vi "_Main_ByRuns_DAC2022_V1.0.vi"() -> ()   [LabVIEW 2017]
uses:
  <vilib>/Instr/_visa.llb/VISA Configure Serial Port (Instr).vi
panel:
  out "Field, kV/cm":dbl
  out "Current, mA":dbl
  out "Voltage, V":dbl
  in  "COM DAC":refnum<visa-resource-name>
  in  "WaveForm":i32(listbox)
  in  "Auto\nturn OFF":bool
  in  "Content":i32(listbox)
  out "LastTrigTimer, s":dbl
  in  "Graph every, cycle":dbl=10.0 min=1.0 max=100.0
  in  "SendPeriod, ms":dbl=100.0 min=10.0 max=10000.0
  out "RunsNeed":i32
  out "Time LOG":cluster{dbl[], dbl[]}(graph)
  out "TrigTimer, s":dbl
  out "Bytes at Port":u32
  out "RecTry":i32
  out "OutVoltage, V":dbl
  in  "Exposition, s":dbl=3.0
  out "Channel 2, V":dbl format="%#_5g"
  out "Channel 1, V":dbl format="%#_5g"
  in  "Stop Button":bool
  in  "Start Button":bool
  in  "Sample H, um":dbl=32.0
  out "VoltageArray, V":dbl[](array[numeric])
  out "Shutter Red":bool
  out "Shutter Green":bool
  in  "Frames In Run":u32=180
  out "Global Frame Done":u32
  out "Now is Run #":u32
  out "Frame In Run Done":u32
  in  "Step, kV/cm":dbl=1.0 min=0.01 max=1000.0
  in  "Amplitude, kV/cm":dbl=10.0 min=10.0 max=1500.0
  in  "LOG file":path
  in  "COM ADC":refnum<visa-resource-name>
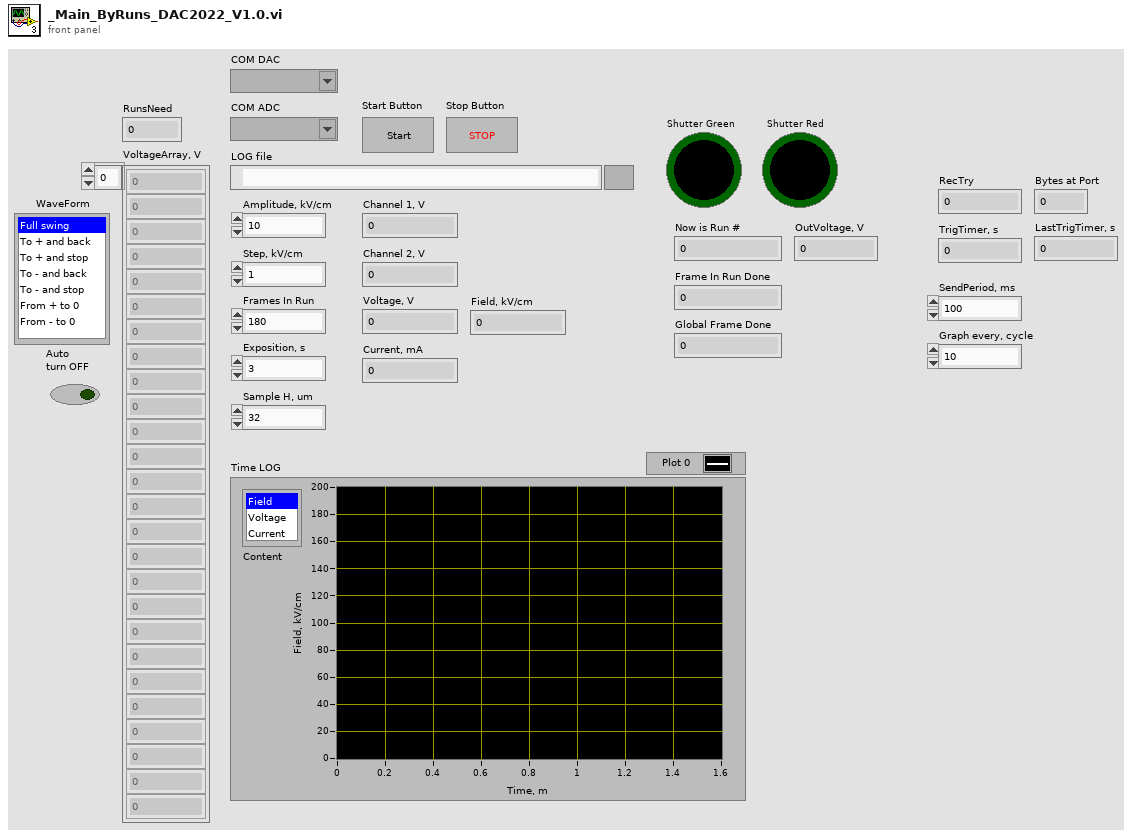
[diagram p1: front panel]
types:
  T1 = cluster{i32, i32, u32, "TrigState":bool, "TrigTimer, s":dbl, "CurrentError":bool}
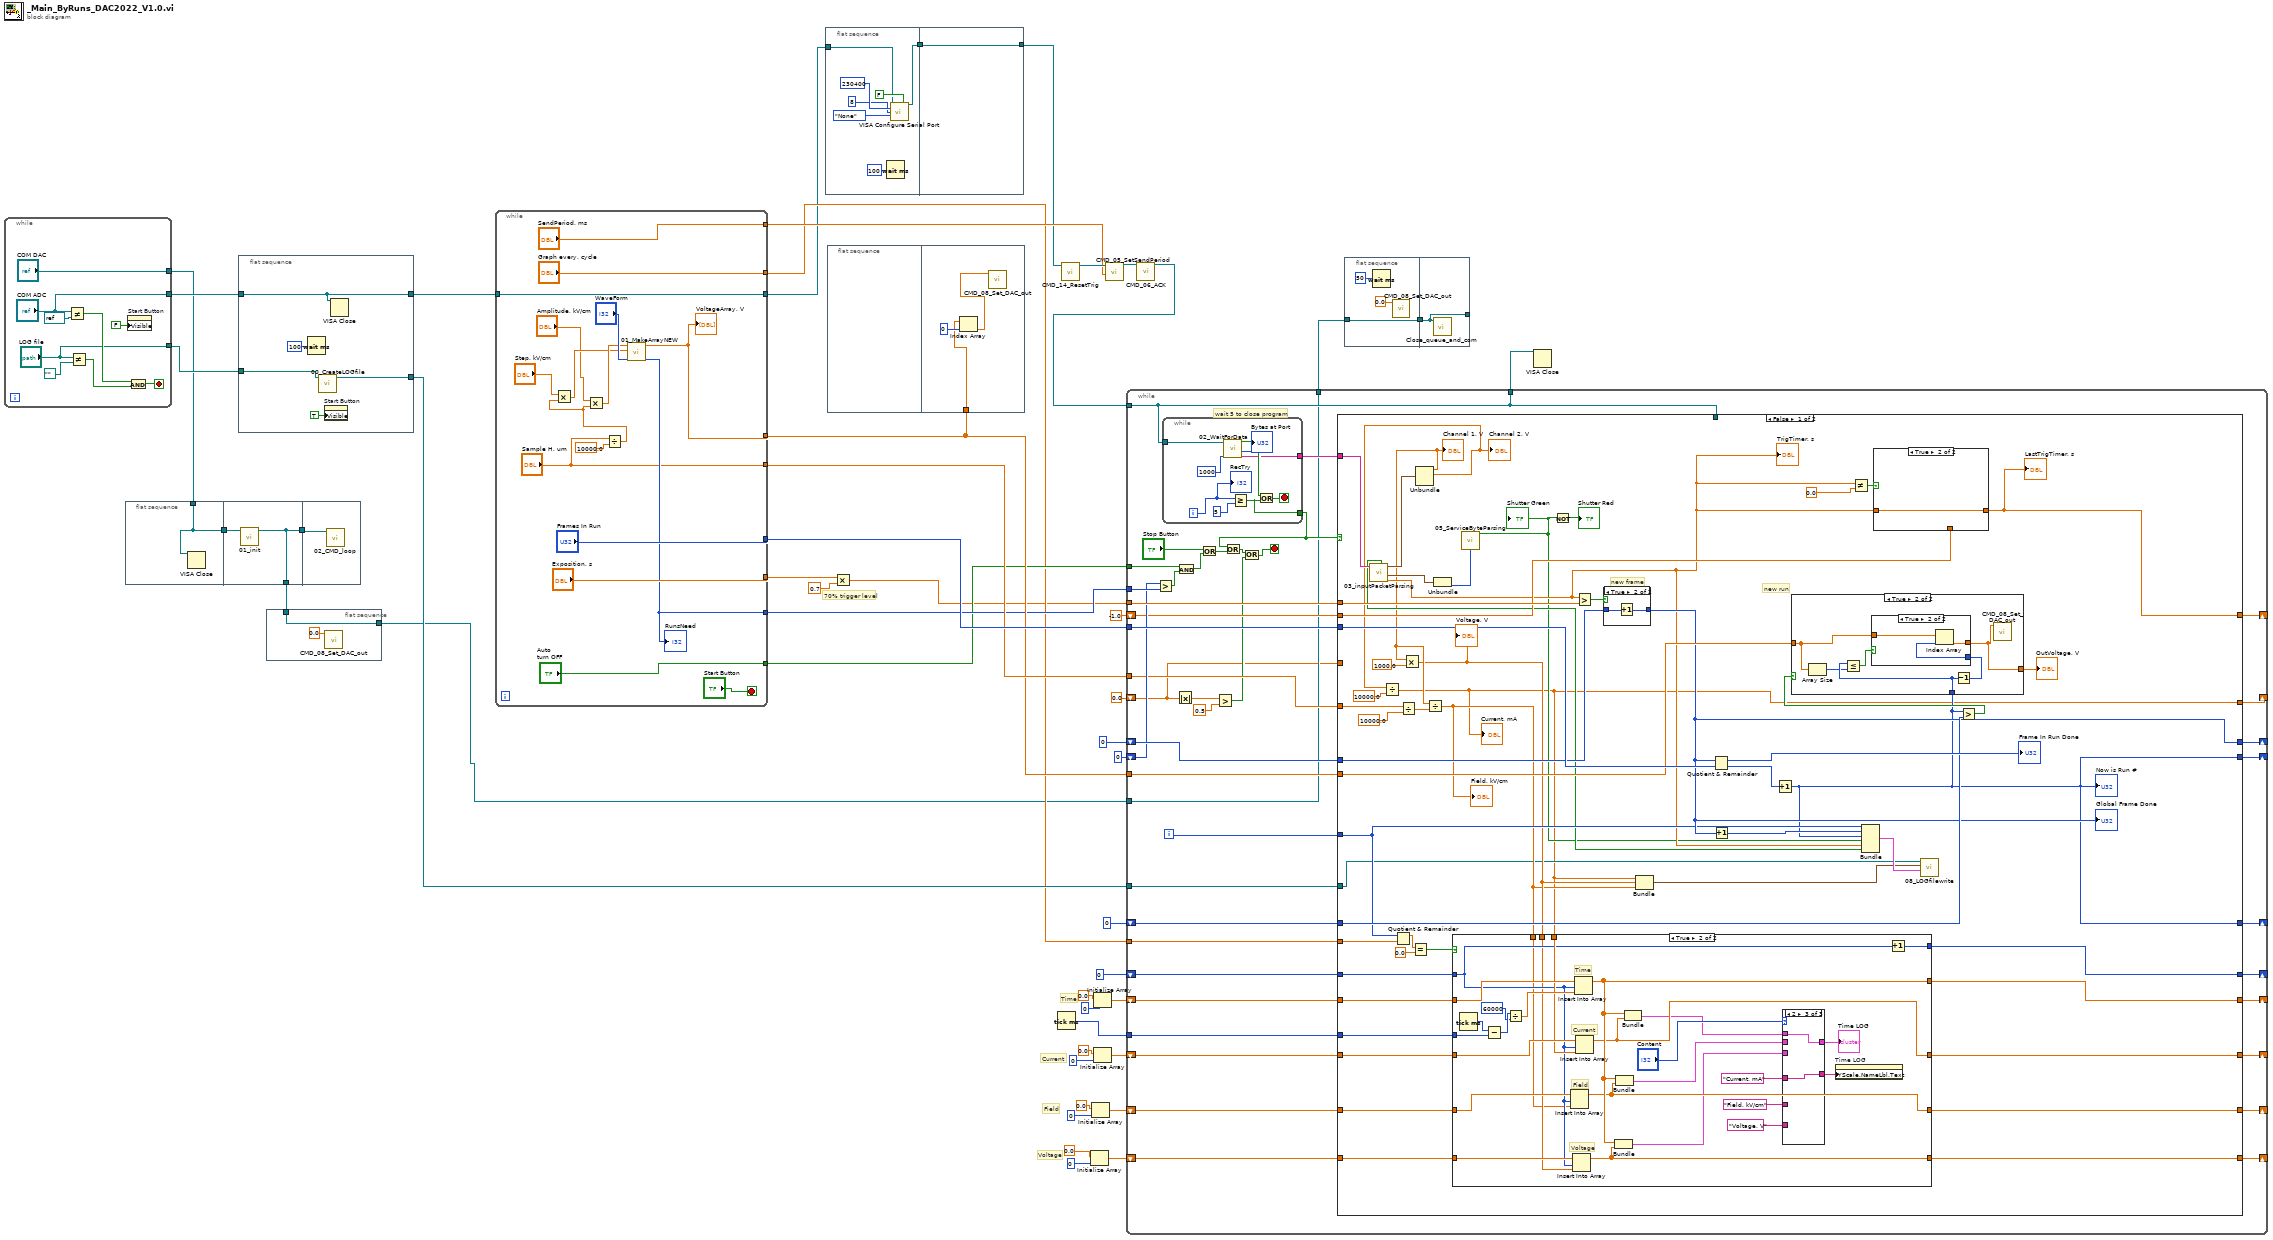
[diagram p0: block diagram]
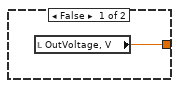
[diagram p6: hidden frame]
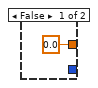
[diagram p7: hidden frame]
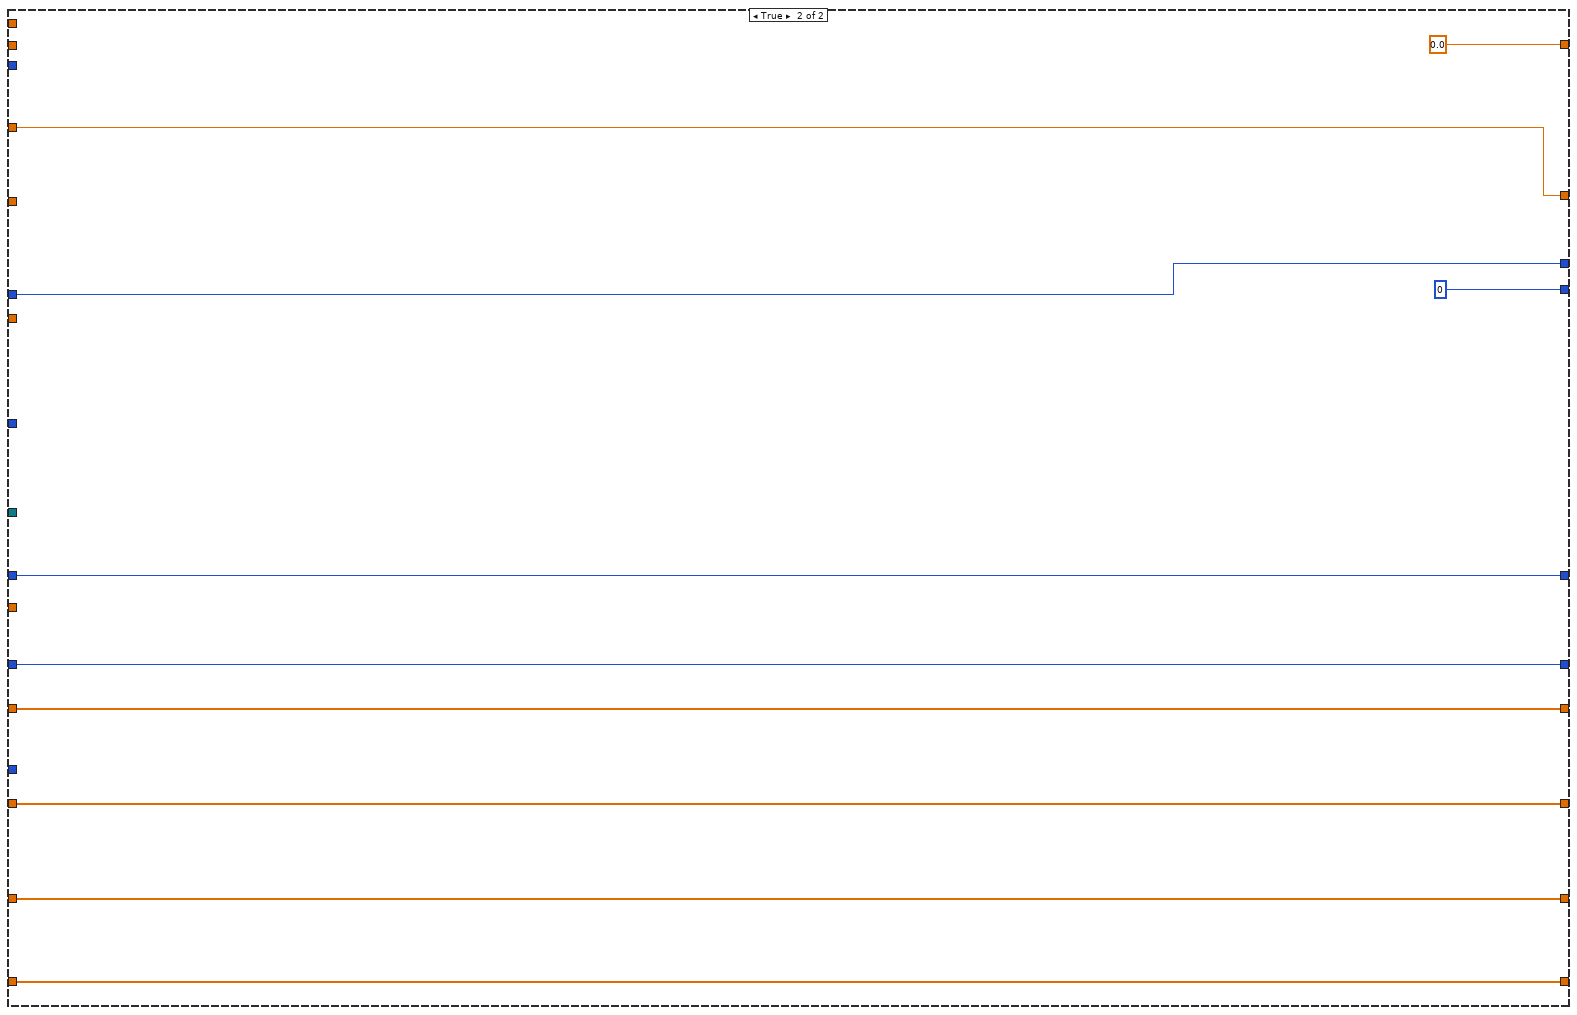
[diagram p9: hidden frame]
diagram:
  # "70% trigger level"
  # "Voltage"
  # "Field"
  # "Time"
  # "Current"
  n1 = while {
    tunnel: ["COM ADC"] -> w15
    tunnel: ["LOG file"] -> w14
    tunnel: ["COM DAC"] -> w6
    stop <- w54 stop-if-true
    n2 = Not Equal?(x="COM ADC", y=refnum<visa-resource-name> refnum ("COM port")) -> (x != y?=w51:bool)
    n3 = Not Equal?(x="LOG file", y=path "" ("LOG file")) -> (x != y?=w52:bool)
    n4 = property on="Start Button" class="Bool"("Visible"=FALSE) -> ()  [unwired: 2 in, 2 out]
    n5 = And(x=w51, y=w52) -> (x .and. y?=w54:bool)
  }
  n6 = flat-sequence {
    tunnel: [w57] -> w8
    tunnel: w6 -> [w57]
    tunnel: w8 -> [w59]
    tunnel: [w58] -> w5
    tunnel: [w58] -> w7
    tunnel: w7 -> [w60]
    frame #0 {
      n7 = VISA Close(VISA resource name=w57) -> ()  [unwired: 1 in, 1 out]
    }
    frame #1 {
      n8 = call "01_init.vi"("COM port"=w59) -> ("VISA resource name out"=w58:refnum<visa-resource-name>)  [unwired: 8 in, 2 out]
    }
    frame #2 {
      n9 = call "02_CMD_loop.vi"("VISA resource name"=w60) -> ()  [unwired: 11 in]
    }
  }
  n10 = flat-sequence {
    tunnel: [w65] -> w45
    tunnel: w15 -> [w61]
    tunnel: w14 -> [w62]
    tunnel: [w61] -> w13
    frame #0 {
      n11 = Wait (ms)(milliseconds to wait=u32 100) -> ()  [unwired: 1 out]
      n12 = call "00_CreateLOGfile.vi"("LOG file"=w62) -> ("refnum out"=w65:refnum<file>)  [unwired: 10 in]
      n13 = property on="Start Button" class="Bool"("Visible"=TRUE) -> ()  [unwired: 2 in, 2 out]
      n14 = VISA Close(VISA resource name=w61) -> ()  [unwired: 1 in, 1 out]
    }
  }
  n15 = flat-sequence {
    tunnel: w5 -> [w66]
    tunnel: [w66] -> w2
    frame #0 {
      n16 = call "CMD_08_Set_DAC_out.vi"("DAC voltage, V"=0.0) -> ()  [unwired: 11 in]
    }
  }
  n17 = while {
    tunnel: w13 -> [w77]
    tunnel: [w77] -> w11
    tunnel: [w76] -> w39
    tunnel: ["Sample H, um"] -> w46
    tunnel: ["Frames In Run"] -> w47
    tunnel: ["Exposition, s"] -> w24
    tunnel: [w75] -> w30
    tunnel: ["Auto\nturn OFF"] -> w28
    tunnel: ["SendPeriod, ms"] -> w27
    tunnel: ["Graph every, cycle"] -> w26
    stop <- "Start Button" stop-if-true
    n18 = Divide(x="Sample H, um", y=10000.0) -> (x/y=w69:dbl)
    n19 = Multiply(x="Step, kV/cm", y=w69) -> (x*y=w71:dbl)
    n20 = Multiply(x="Amplitude, kV/cm", y=w69) -> (x*y=w72:dbl)
    n21 = call "01_MakeArrayNEW.vi"("Amp"=w72, "Step"=w71, "WaveForm"="WaveForm") -> ("Array"=w76:dbl[], "ArraySize"=w75:i32)  [unwired: 6 in]
    "VoltageArray, V" <- w76
    "RunsNeed" <- w75
  }
  n22 = flat-sequence {
    tunnel: w11 -> [w87]
    tunnel: [w86] -> w12
    tunnel: w12 -> [w92]
    tunnel: [w92] -> w10
    frame #0 {
      n23 = Wait (ms)(milliseconds to wait=u32 100) -> ()  [unwired: 1 out]
      n24 = call-poly "VISA Configure Serial Port"("VISA resource name"=w87, "Enable Termination\nChar (T)"=FALSE ("Enable Termination\nChar (T)"), "baud rate (9600)"=u32 230400, "data bits (8)"=u16 8, "parity (0:none)"=enum16{"None", "Odd", "Even", "Mark", "Space"}."None") -> ("VISA resource name out"=w86:refnum<visa-resource-name>)  [unwired: 9 in, 1 out]
    }
    frame #1 {
    }
  }
  n25 = flat-sequence {
    tunnel: w39 -> [w94]
    frame #0 {
    }
    frame #1 {
      n26 = Index Array(array=w94, index=0) -> (element=w93:dbl)
      n27 = call "CMD_08_Set_DAC_out.vi"("DAC voltage, V"=w93) -> ()  [unwired: 11 in]
    }
  }
  n28 = Multiply(x=w24, y=0.7) -> (x*y=w25:dbl)
  n29 = Tick Count (ms)() -> (millisecond timer value=w34:u32)
  n30 = call "CMD_14_ResetTrig.vi"("VISA resource name"=w10) -> ("VISA resource name out"=w42:refnum<visa-resource-name>)  [unwired: 10 in]
  n31 = Initialize Array(0.0 ("element"), 0 ("dimension size")) -> (w16:dbl[])
  n32 = Initialize Array(0.0 ("element"), 0 ("dimension size")) -> (w17:dbl[])
  n33 = Initialize Array(0.0 ("element"), 0 ("dimension size")) -> (w31:dbl[])
  n34 = Initialize Array(0.0 ("element"), 0 ("dimension size")) -> (w35:dbl[])
  n35 = call "CMD_05_SetSendPeriod.vi"("Period, ms"=w27, "VISA resource name"=w42) -> ("VISA resource name out"=w41:refnum<visa-resource-name>)  [unwired: 9 in]
  n36 = call "CMD_06_ACK.vi"("VISA resource name"=w41) -> ("VISA resource name out"=w40:refnum<visa-resource-name>)  [unwired: 10 in]
  n37 = while {
    tunnel: w40 -> [w104]
    tunnel: w39 -> [w128]
    tunnel: w47 -> [w134]
    tunnel: w25 -> [w136]
    tunnel: w46 -> [w105]
    tunnel: w45 -> [w135]
    shift-right: [w131] -> _
    shift-left: 0 -> [w133]
    shift-right: [w130] -> _
    shift-left: u32 0 -> [w129]
    shift-right: [w126] -> _
    shift-left: 0 -> [w127]
    tunnel: w34 -> [w124]
    shift-right: [w122] -> _
    shift-left: w35 -> [w125]
    shift-right: [w121] -> _
    shift-left: w31 -> [w123]
    tunnel: w30 -> [w117]
    shift-right: [w119] -> _
    shift-left: u32 0 -> [w116]
    tunnel: w28 -> [w113]
    tunnel: w26 -> [w112]
    shift-right: [w111] -> _
    shift-left: -1.0 ("TrigTimer, s") -> [w110]
    shift-right: [w107] -> _
    shift-left: w17 -> [w109]
    shift-right: [w106] -> _
    shift-left: w16 -> [w108]
    tunnel: [w103] -> w3
    tunnel: [w104] -> w9
    tunnel: w2 -> [w103]
    shift-right: [w102] -> _
    shift-left: 0.0 -> [w96]
    i -> [w132]
    stop <- w100 stop-if-true
    # "wait 5 to close program"
    n38 = Greater?(x=w116, y=w117) -> (0:w114:bool)
    n39 = while {
      tunnel: w104 -> [w257]
      tunnel: [w260] -> w138
      tunnel: [w261] -> w137
      i -> [w259]
      stop <- w263 stop-if-true
      n40 = call "02_WaitForData.vi"("WaitTimeoutMS"=u32 1000, "VISA"=w257) -> ("Buffer"=w261:string, "Bytes at Port"=→"Bytes at Port":u32, "Data Recived"=w262:bool)  [unwired: 7 in]
      n41 = Greater Or Equal?(x=w259, y=5) -> (x >= y?=w260:bool)
      n42 = Or(x=w262, y=w260) -> (x .or. y?=w263:bool)
      "RecTry" <- w259
    }
    n43 = Absolute Value(x=w96) -> (abs(x)=w97:dbl)
    n44 = And(x=w113, y=w114) -> (x .and. y?=w115:bool)
    n45 = Or(x="Stop Button", y=w115) -> (x .or. y?=w120:bool)
    n46 = Greater?(x=w97, y=0.5) -> (0:w98:bool)
    n47 = Or(x=w138, y=w120) -> (x .or. y?=w99:bool)
    n48 = Or(x=w99, y=w98) -> (x .or. y?=w100:bool)
    n49 = case shown="False" w138 {
      tunnel: w137 -> [w192 _]
      tunnel: w136 -> [w188 _]
      tunnel: w135 -> [w140 _]
      tunnel: w134 -> [w189 _]
      tunnel: w133 -> [w186 w256]
      tunnel: w132 -> [w173 _]
      tunnel: [w178 w256] -> w131
      tunnel: [w164 w255] -> w130
      tunnel: w129 -> [w181 w255]
      tunnel: w128 -> [w182 _]
      tunnel: w104 -> [_ _]
      tunnel: w127 -> [w171 w254]
      tunnel: [w170 w254] -> w126
      tunnel: w125 -> [w169 w253]
      tunnel: w124 -> [w168 _]
      tunnel: w123 -> [w167 w252]
      tunnel: [w166 w253] -> w122
      tunnel: [w165 w252] -> w121
      tunnel: [w164 u32 0] -> w119
      tunnel: w112 -> [w163 _]
      tunnel: [w160 0.0 ("TrigTimer, s")] -> w111
      tunnel: w110 -> [w159 _]
      tunnel: w109 -> [w155 w249]
      tunnel: w108 -> [w154 w248]
      tunnel: [w153 w249] -> w107
      tunnel: [w152 w248] -> w106
      tunnel: w105 -> [w146 _]
      tunnel: [w139 w247] -> w102
      tunnel: w96 -> [_ w247]
      frame False {
        # "new run"
        # "new frame"
        n50 = call "03_inputPacketParsing.vi"("string"=w192) -> ("TrigTimer, s"=w158:dbl, "Service state"=w177:cluster{u8, u8}, "Voltage"=w190:cluster{dbl, dbl, dbl, dbl}, "CurrentError"=w157:bool)  [unwired: 6 in, 1 out]
        "TrigTimer, s" <- w158
        n51 = Quotient & Remainder(x=w173, y=w163) -> (x-y*floor(x/y)=w175:dbl)  [unwired: 1 out]
        n52 = Divide(x=w146, y=10000.0) -> (x/y=w147:dbl)
        n53 = Equal?(x=w175, y=0.0) -> (x = y?=w172:bool)
        n54 = Unbundle(w190) -> (w148:dbl, w150:dbl)  [unwired: 2 out]
        "Channel 1, V" <- w148
        "Channel 2, V" <- w150
        n55 = Divide(x=w150, y=10000.0) -> (x/y=w139:dbl)
        "Current, mA" <- w139
        n56 = Multiply(x=w148, y=1000.0) -> (x*y=w143:dbl)
        "Voltage, V" <- w143
        n57 = Divide(x=w148, y=w147) -> (x/y=w142:dbl)
        "Field, kV/cm" <- w142
        n58 = Unbundle(w177) -> (w176:u8)  [unwired: 1 out]
        n59 = case shown="True" w172 {
          tunnel: w171 -> [w199 w215]
          tunnel: [w199 w222] -> w170
          tunnel: w169 -> [w197 w220]
          tunnel: w168 -> [_ w225]
          tunnel: w167 -> [w198 w219]
          tunnel: [w198 w211] -> w165
          tunnel: [w197 w214] -> w166
          tunnel: w139 -> [_ w218]
          tunnel: w155 -> [w196 w217]
          tunnel: w154 -> [w195 w216]
          tunnel: [w196 w212] -> w153
          tunnel: [w195 w213] -> w152
          tunnel: w143 -> [_ w201]
          tunnel: w142 -> [_ w200]
          frame False {
          }
          frame True {
            # "Time"
            # "Voltage"
            # "Field"
            # "Current"
            n60 = Tick Count (ms)() -> (millisecond timer value=w226:u32)
            n61 = Subtract(x=w226, y=w225) -> (x-y=w224:u32)
            n62 = Divide(x=w224, y=u32 60000) -> (x/y=w221:dbl)
            n63 = Insert Into Array(array=w217, index=w215, new element=w200) -> (w212:dbl[])
            n64 = Insert Into Array(array=w216, index=w215, new element=w201) -> (w213:dbl[])
            n65 = Insert Into Array(array=w220, index=w215, new element=w221) -> (w214:dbl[])
            n66 = Insert Into Array(array=w219, index=w215, new element=w218) -> (w211:dbl[])
            n67 = Bundle(w214, w213) -> (w207:cluster{dbl[], dbl[]})  [unwired: 1 in]
            n68 = Bundle(w214, w212) -> (w208:cluster{dbl[], dbl[]})  [unwired: 1 in]
            n69 = Bundle(w214, w211) -> (w209:cluster{dbl[], dbl[]})  [unwired: 1 in]
            n70 = case shown="2" "Content" {
              tunnel: w209 -> [_ _ w232]
              tunnel: w208 -> [w228 _ _]
              tunnel: w207 -> [_ w230 _]
              tunnel: [w228 w230 w232] -> w206
              tunnel: "Current, mA" ("Y Scale.Name Label.Text") -> [_ _ w231]
              tunnel: "Field, kV/cm" ("Y Scale.Name Label.Text") -> [w227 _ _]
              tunnel: "Voltage, V" ("Y Scale.Name Label.Text") -> [_ w229 _]
              tunnel: [w227 w229 w231] -> w202
              frame 0, Default {
              }
              frame 1 {
              }
              frame 2 {
              }
            }
            "Time LOG" <- w206
            n71 = property on="Time LOG" class="XYGraph (strict)"("YScale.NameLbl.Text"=w202) -> ()  [unwired: 2 in, 2 out]
            n72 = Increment(x=w215) -> (x+1=w222:i32)
          }
        }
        n73 = call "05_ServiceByteParsing.vi"("InputByte"=w176) -> ("TrigState"=w156:bool)  [unwired: 7 in, 3 out]
        "Shutter Green" <- w156
        n74 = Not(x=w156) -> (.not. x?=→"Shutter Red":bool)
        n75 = Greater?(x=w158, y=w188) -> (0:w187:bool)
        n76 = case shown="True" w187 {
          tunnel: w186 -> [w244 w246]
          tunnel: [w244 w245] -> w178
          frame False {
          }
          frame True {
            n77 = Increment(x=w246) -> (x+1=w245:i32)
          }
        }
        "Global Frame Done" <- w178
        n78 = Bundle(w139, w143, w142) -> (w141:cluster{dbl, dbl, dbl})  [unwired: 1 in]
        n79 = Quotient & Remainder(x=w178, y=w189) -> (x-y*floor(x/y)=→"Frame In Run Done":u32, floor(x/y)=w184:u32)
        n80 = Increment(x=w178) -> (x+1=w179:i32)
        n81 = Increment(x=w184) -> (x+1=w164:u32)
        "Now is Run #" <- w164
        n82 = Not Equal?(x=w158, y=0.0) -> (x != y?=w162:bool)
        n83 = Bundle(w173, w179, w164, "TrigState"=w156, "TrigTimer, s"=w158, "CurrentError"=w157) -> (w144:T1)  [unwired: 1 in]
        n84 = case shown="True" w162 {
          tunnel: [w193 w194] -> w160
          tunnel: w158 -> [_ w194]
          tunnel: w159 -> [w193 _]
          frame False {
          }
          frame True {
          }
        }
        "LastTrigTimer, s" <- w160
        n85 = call "08_LOGfilewrite.vi"("Counters"=w144, "output cluster"=w141, "refnum out"=w140) -> ()  [unwired: 9 in]
        n86 = Greater?(x=w164, y=w181) -> (0:w185:bool)
        n87 = case shown="True" w185 {
          tunnel: w182 -> [_ w235]
          tunnel: w164 -> [_ w238]
          tunnel: [w233 w234] -> w180
          frame False {
            n88 = local read "OutVoltage, V"() -> (w233:dbl)
          }
          frame True {
            n89 = Array Size(array=w235) -> (size(s)=w237:i32)
            n90 = Less Or Equal?(x=w238, y=w237) -> (x <= y?=w236:bool)
            n91 = Decrement(x=w238) -> (x-1=w239:u32)
            n92 = case shown="True" w236 {
              tunnel: w239 -> [_ w243]
              tunnel: w235 -> [_ w242]
              tunnel: [0.0 w241] -> w234
              frame False {
              }
              frame True {
                n93 = Index Array(array=w242, index=w243) -> (element=w241:dbl)
              }
            }
            n94 = call "CMD_08_Set_DAC_out.vi"("DAC voltage, V"=w234) -> ()  [unwired: 11 in]
          }
        }
        "OutVoltage, V" <- w180
      }
      frame True {
      }
    }
  }
  n95 = flat-sequence {
    tunnel: w3 -> [w267]
    tunnel: [w267] -> w4
    tunnel: [w269] -> _
    tunnel: w4 -> [w269]
    frame #0 {
      n96 = Wait (ms)(milliseconds to wait=u32 50) -> ()  [unwired: 1 out]
      n97 = call "CMD_08_Set_DAC_out.vi"("DAC voltage, V"=0.0) -> ()  [unwired: 11 in]
    }
    frame #1 {
      n98 = call "Close_queue_and_com.vi"("VISA"=w269) -> ()  [unwired: 11 in]
    }
  }
  n99 = VISA Close(VISA resource name=w9) -> ()  [unwired: 1 in, 1 out]
